vi "HAL camera program for acquisition.vi"(2 "error in":errorcluster, 3 "Camera Parameters (important)":T1={"Exposure Time (sec)"=0.0, "EM CCD Gain"=0, "Readout Settings"={"Clocking mode"=0, "Speed"=0, "Clear mode"=2, "# clear cycles"=0, "ADC Gain"=0}, "Image Size"={"H Bin"=0, "V Bin"=0, "Left"=0, "Top"=0, "Right"=0, "Bottom"=0}} {"Readout Settings"."ADC Gain" min=-1 step=1; "Readout Settings"."Clear mode" items=["Don't clear", "Clear pre-exposure", "Clear pre-sequence", "Clear post-sequence", "Clear pre- and post-sequence", "Clear pre-exposure and post-sequence"]; "Readout Settings"."Speed" items=["1 Mhz, no EM", "5 Mhz, no EM", "5 Mhz, EM", "10 MHz, EM"]; "Readout Settings"."Clocking mode" items=["Normal", "Frame-transfer"]; "EM CCD Gain" scale=0.01..4096.0; "Exposure Time (sec)" scale=0.001..10.0 scale format="%#_1g"}) -> (0 "error out":errorcluster, 1 "Actual Exposure Time (sec)":sgl)   [LabVIEW 2011]
uses:
  Camera/camera globals.vi
  cascade readout settings.ctl
  HAL camera parameters important.ctt
  Camera/Image size.ctt
panel:
  # "Camera: Roper Cascade"
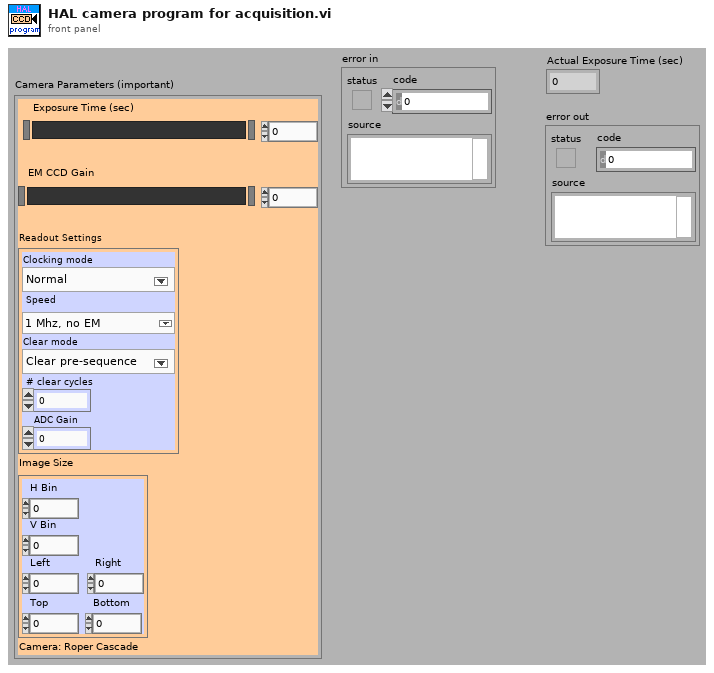
[diagram p1: front panel]
types:
  T1 = typedef "HAL camera parameters important.ctt" = cluster{"Exposure Time (sec)":sgl, "EM CCD Gain":u16, "Readout Settings":T2, "Image Size":T3}
  T2 = typedef "cascade readout settings.ctl" = cluster{"Clocking mode":u8, "Speed":u16, "Clear mode":u8, "# clear cycles":u16, "ADC Gain":i32}
  T3 = typedef "Image size.ctt" = cluster{"H Bin":i32, "V Bin":i32, "Left":i32, "Top":i32, "Right":i32, "Bottom":i32}
  T4 = cluster{"X Start":u32, "X End":u32, "X Bin":u32, "Y Start":u32, "Y End":u32, "Y Bin":u32}
  T5 = cluster{"Clear mode":u8, "# clear cycles":u16, "Clocking mode":u8}
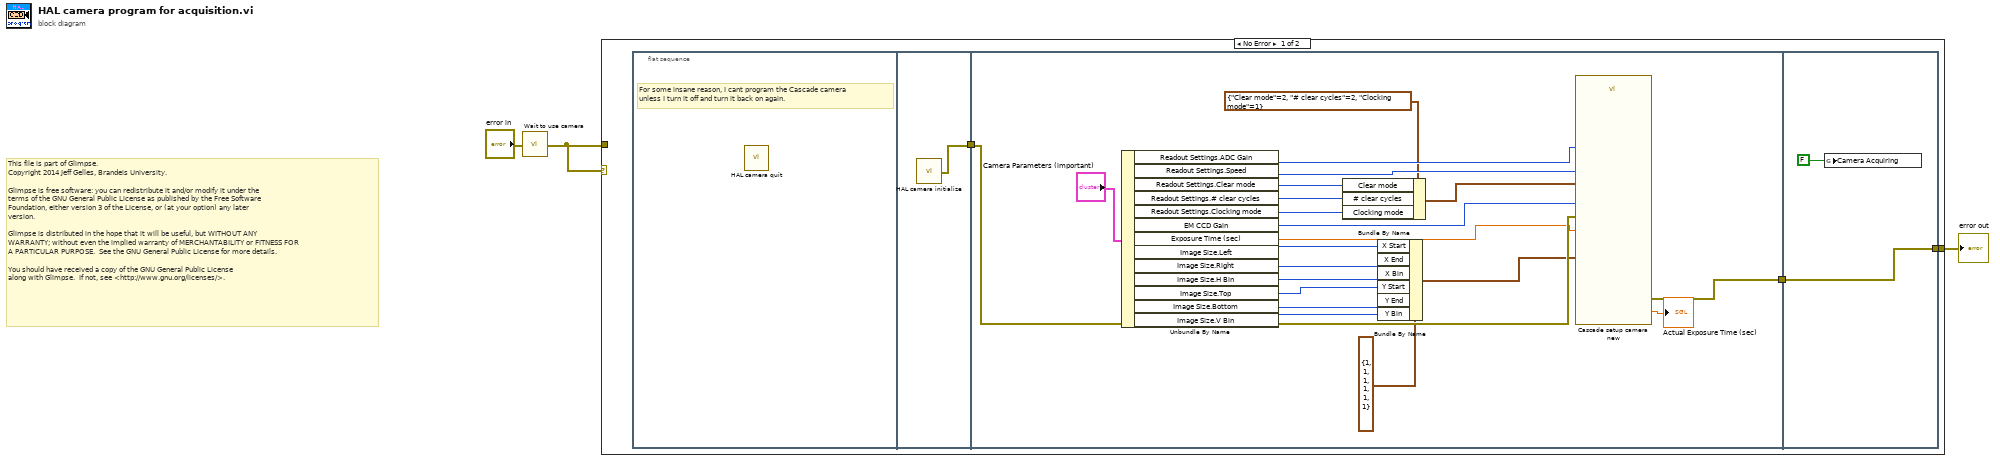
[diagram p0: block diagram]
diagram:
  # "This file is part of Glimpse. \nCopyright 2014 Jeff Gelles, Brandeis University.    \n\nGlimpse is free software: you can redistribute it and/or modify it under the \nterms of the GNU General Public License as published by the Free Software \nFoundation, either version 3 of the License, or (at your option) any later \nversion.\n\nGlimpse is distributed in the hope that it will be useful, but WITHOUT ANY \nWARRANTY; without even the implied warranty of MERCHANTABILITY or FITNESS FOR \nA PARTICULAR PURPOSE.  See the GNU General Public License for more details.\n\nYou should have received a copy of the GNU General Public License\nalong with Glimpse.  If not, see <http://www.gnu.org/licenses/>."
  n1 = call "Wait to use camera.vi"("error in"="error in") -> ("error out"=w1:errorcluster)
  n2 = case shown="No Error" w1 {
    tunnel: [w6 w31] -> w3
    tunnel: w1 -> [_ w31]
    frame No Error {
      n3 = flat-sequence {
        tunnel: [w7] -> w4
        tunnel: [w9] -> w5
        tunnel: w4 -> [w19]
        tunnel: [w29] -> w6
        tunnel: w5 -> [w29]
        frame #0 {
          # "For some insane reason, I cant program the Cascade camera\nunless I turn it off and turn it back on again."
          n4 = call "HAL camera quit.vi"() -> ()  [unwired: 1 out]
        }
        frame #1 {
          n5 = call "HAL camera initialize.vi"() -> ("error out"=w7:errorcluster)
        }
        frame #2 {
          n6 = Unbundle By Name("Camera Parameters (important)") -> ("Readout Settings.ADC Gain"=w27:i32, "Readout Settings.Speed"=w26:u16, "Readout Settings.Clear mode"=w23:u8, "Readout Settings.# clear cycles"=w22:u16, "Readout Settings.Clocking mode"=w21:u8, "EM CCD Gain"=w20:u16, "Exposure Time (sec)"=w18:sgl, "Image Size.Left"=w15:i32, "Image Size.Right"=w14:i32, "Image Size.H Bin"=w13:i32, "Image Size.Top"=w12:i32, "Image Size.Bottom"=w11:i32, "Image Size.V Bin"=w10:i32)
          n7 = Bundle By Name(cluster=T5 {"Clear mode"=2, "# clear cycles"=2, "Clocking mode"=1} ("Clocking parameters"), "Clear mode"=w23, "# clear cycles"=w22, "Clocking mode"=w21) -> (w25:T5)
          n8 = Bundle By Name(cluster=T4 {"X Start"=1, "X End"=1, "X Bin"=1, "Y Start"=1, "Y End"=1, "Y Bin"=1} ("ROI"), "X Start"=w15, "X End"=w14, "X Bin"=w13, "Y Start"=w12, "Y End"=w11, "Y Bin"=w10) -> (w16:T4)
          n9 = call "Cascade setup camera new.vi"("ADC speed"=w26, "Exposure"=w18, "Clocking parameters"=w25, "ADC Gain"=w27, "error in (no error)"=w19, "EM Gain"=w20, "ROI"=w16) -> (8:→"Actual Exposure Time (sec)":dbl, "error out (no error)"=w9:errorcluster)  [unwired: 2 in, 5 out]
        }
        frame #3 {
          n10 = global write "camera globals.vi" "Camera Acquiring"(FALSE ("Andor Aquiring")) -> ()
        }
      }
    }
    frame Error {
    }
  }
  "error out" <- w3
